vi "Drive Motors.vi"() -> ()   [LabVIEW 2018]
uses:
  <vilib>/Rock Robotics/WPI/ThirdParty/Phoenix-LabVIEW/Motor Controller/Controls/CTRE_Phoenix_MotorControl_ControlMode.ctl
  <vilib>/Rock Robotics/WPI/ThirdParty/Phoenix-LabVIEW/Motor Controller/Controls/CTRE_Phoenix_MotorControl_NeutralMode.ctl
  Framework/Robot Global Data.vi
  <vilib>/Rock Robotics/WPI/ThirdParty/Phoenix-LabVIEW/Motor Controller/Get/CTRE_Phoenix_MotorController_GetOutputCurrent_Enhanced.vi
  <vilib>/ptbypt/NI_PtbyPt.lvlib
panel:
  out "Peak Current":dbl[](array[numeric])
  in  "Target Time (s)":dbl=0.25
  in  "dropout speed":dbl=0.3
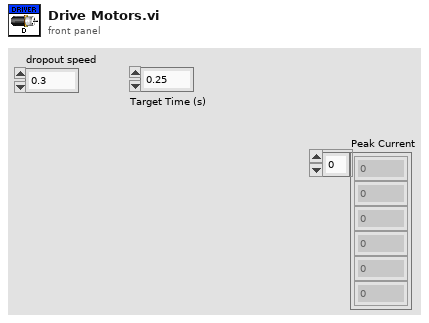
[diagram p1: front panel]
types:
  T1 = typedef "CTRE_Phoenix_MotorControl_NeutralMode.ctl" = enum8{"EEPROMSetting", "Override to Coast", "Override to Brake"}
  T2 = typedef "WPI_MotorControlDeviceRef.ctl" = cluster{"DeviceStatus":errorcluster, "Type":T3, "PWM":cluster{"PWM Channel":T4, "DeadBand":T5}, "CAN":cluster{"Device Number":u8, "SetOutput VI Ref":variant, "GetOutput VI Ref":variant, "Enable VI Ref":variant, "Disable VI Ref":variant, "Data":variant}, "Invert":bool, "DIO PWM":cluster{"PWM \"Enable\" Channel":T4, "DIOChannel":T6, "PWM Rate":dbl}}
  T3 = typedef "WPI_MotorControlType.ctl" = enum16{"PWM", "CAN", "DIO PWM"}
  T4 = typedef "FPGA_DIOPWMChannel.ctl" = enum8{"PWM 0", "PWM 1", "PWM 2", "PWM 3", "PWM 4", "PWM 5", "PWM 6", "PWM 7", "PWM 8", "PWM 9", "PWM MXP 0", "PWM MXP 1", "PWM MXP 2", "PWM MXP 3", "PWM MXP 4", "PWM MXP 5", "PWM MXP 6", "PWM MXP 7", "PWM MXP 8", "PWM MXP 9", "Invalid"}
  T5 = typedef "WPI_PWMDeadband.ctl" = cluster{"Name":string, "maxPositivePwm":i32, "minPositivePwm":i32, "centerPwm":i32, "maxNegativePwm":i32, "minNegativePwm":i32, "angularRange":u16}
  T6 = typedef "FPGA_DIOChannel.ctl" = enum8{"DIO 0", "DIO 1", "DIO 2", "DIO 3", "DIO 4", "DIO 5", "DIO 6", "DIO 7", "DIO 8", "DIO 9", "DIO MXP 0", "DIO MXP 1", "DIO MXP 2", "DIO MXP 3", "DIO MXP 4", "DIO MXP 5", "DIO MXP 6", "DIO MXP 7", "DIO MXP 8", "DIO MXP 9", "DIO MXP 10", "DIO MXP 11", "DIO MXP 12", "DIO MXP 13", "DIO MXP 14", "DIO MXP 15", "SPI Port CS1", "SPI Port CS2", "SPI Port CS3", "SPI Port MISO", "SPI Port MOSI", "Invalid"}
  T7 = typedef "CTRE_Phoenix_MotorControl_ControlMode.ctl" = u16
  T8 = typedef "WPI_DriverStationRobotMode2.ctl" = enum16{"Autonomous Disabled", "Autonomous Enabled", "Teleop Disabled", "Teleop Enabled", "Disconnected", "Finish", "Test Disabled", "Test Enabled", "Emergency Stopped"}
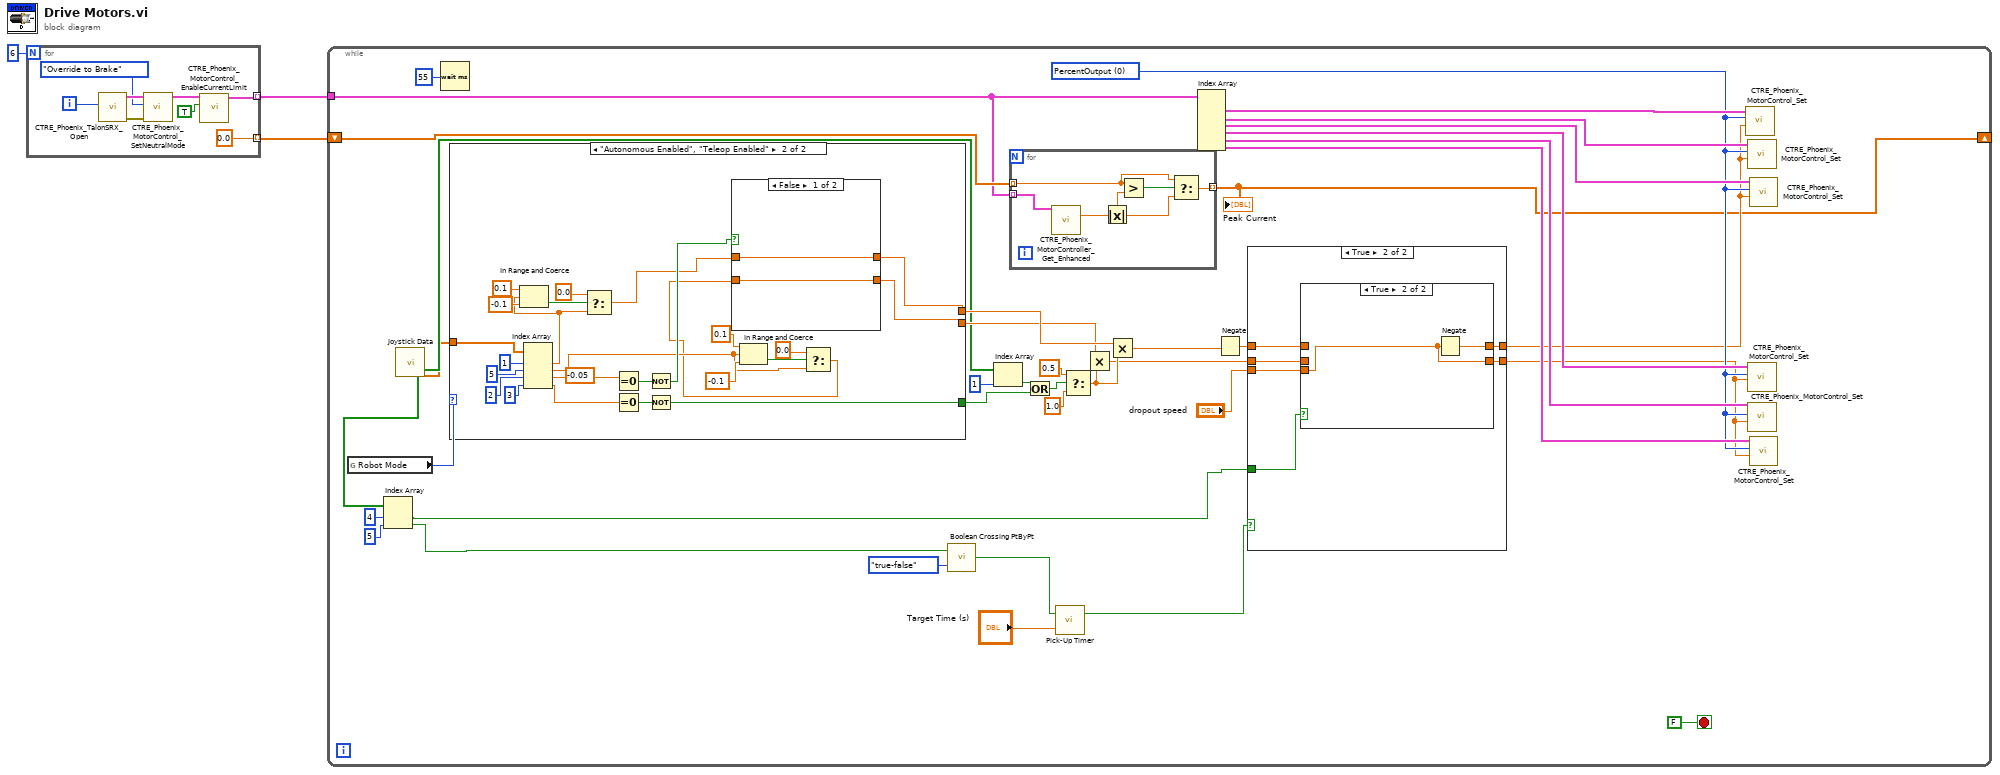
[diagram p0: block diagram]
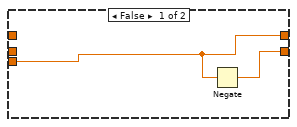
[diagram p2: hidden frame]
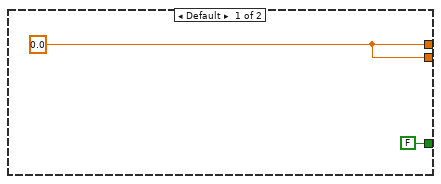
[diagram p4: hidden frame]
diagram:
  n1 = for {
    N: 6 -> [_]
    tunnel: [w6] -> w2 mode=indexing
    tunnel: [0.0] -> w1 mode=indexing
    i -> [w11]
    n2 = call <vilib>:"CTRE_Phoenix_TalonSRX_Open.vi"("Device Number"=w11) -> ("error out"=w10:errorcluster, "CAN Talon SRX Ref"=w9:T2)  [unwired: 9 in]
    n3 = call <vilib>:"CTRE_Phoenix_MotorControl_SetNeutralMode.vi"("error in (no error)"=w10, "Motor Control Neutral Mode"=CTRE_Phoenix_MotorControl_NeutralMode."Override to Brake", "PhoenixMotorControlDevRef"=w9) -> ("PhoenixMotorControlDevRef"=w7:T2)  [unwired: 7 in, 1 out]
    n4 = call <vilib>:"CTRE_Phoenix_MotorControl_EnableCurrentLimit.vi"("Enable Current Limit?"=TRUE, "PhoenixMotorControlDevRef"=w7) -> ("PhoenixMotorControlDevRef"=w6:T2)  [unwired: 8 in, 1 out]
  }
  n5 = while {
    tunnel: w2 -> [w12]
    shift-right: [w18] -> _
    shift-left: w1 -> [w19]
    stop <- FALSE stop-if-true
    w34 = T7 0 items=["PercentOutput"=0, "Position"=1, "Velocity"=2, "Current"=3, "Follower"=5, "MotionProfile"=6, "MotionMagic"=7, "MotionProfileArc"=10, "Disabled"=15] ("Control Mode")
    n6 = global read "Robot Global Data.vi" "Robot Mode"() -> (w50:T8)
    n7 = call "Joystick Data.vi"() -> ("Xbox 360 Out"=w14:bool[], "Right Buttons Out"=w26:bool[], "Xbox One Joy Out"=w25:dbl[])  [unwired: 12 in, 5 out]
    n8 = Index Array(array=w14, index #1=4 ("index"), index #2=5 ("index")) -> (element #1=w15:bool, element #2=w13:bool)
    n9 = Wait (ms)(milliseconds to wait=u32 55) -> ()  [unwired: 1 out]
    n10 = case shown="\"Autonomous Enabled\", \"Teleop Enabled\"" w50 {
      tunnel: [w70 w95] -> w42
      tunnel: [w70 w94] -> w41
      tunnel: [FALSE w85] -> w33
      tunnel: w25 -> [_ w83]
      frame Default {
        w70 = 0.0
      }
      frame "Autonomous Enabled", "Teleop Enabled" {
        (unwired) -0.05 ("lower limit")
        n11 = Index Array(array=w83, index #1=1 ("index"), index #2=5 ("index"), index #3=2 ("index"), index #4=3 ("index")) -> (element #1=w78:dbl, element #2=w72:dbl, element #3=w88:dbl, element #4=w86:dbl)
        n12 = In Range and Coerce(upper limit=0.1, x=w78, lower limit=-0.1) -> (In Range?=w80:bool)  [unwired: 1 out]
        n13 = Select(t=0.0, s=w80, f=w78) -> (s? t:f=w77:dbl)
        n14 = Equal To 0?(x=w88) -> (x = 0?=w89:bool)
        n15 = Equal To 0?(x=w86) -> (x = 0?=w87:bool)
        n16 = Not(x=w89) -> (.not. x?=w84:bool)
        n17 = Not(x=w87) -> (.not. x?=w85:bool)
        n18 = In Range and Coerce(upper limit=0.1, x=w72, lower limit=-0.1) -> (In Range?=w74:bool)  [unwired: 1 out]
        n19 = Select(t=0.0, s=w74, f=w72) -> (s? t:f=w71:dbl)
        n20 = case shown="False" w84 {
          tunnel: w71 -> [w97 w98]
          tunnel: [w96 w98] -> w95
          tunnel: [w97 w98] -> w94
          tunnel: w77 -> [w96 _]
          frame False {
          }
          frame True {
          }
        }
      }
    }
    n21 = call <vilib>:"Boolean Crossing PtByPt.vi"("direction"=enum16{"either", "false-true", "true-false"}."true-false", "input"=w13) -> ("crossing"=w22:bool)  [unwired: 1 in]
    n22 = Index Array(array=w26, index=1) -> (element=w32:bool)
    n23 = for {
      tunnel: w12 -> [w56] mode=indexing
      tunnel: w19 -> [w53] mode=indexing
      tunnel: [w51] -> w18 mode=indexing
      n24 = call-poly <vilib>:"CTRE_Phoenix_MotorController_Get_Enhanced.vi"("PhoenixMotorControlDevRef"=w56) -> ("Output Current"=w55:dbl)  [unwired: 12 in, 2 out]
      n25 = Absolute Value(x=w55) -> (abs(x)=w52:dbl)
      n26 = Greater?(x=w53, y=w52) -> (0:w54:bool)
      n27 = Select(t=w53, s=w54, f=w52) -> (s? t:f=w51:dbl)
    }
    "Peak Current" <- w18
    n28 = Or(x=w32, y=w33) -> (x .or. y?=w31:bool)
    n29 = call "Pick-Up Timer.vi"("Target Time (s)"="Target Time (s)", "Reset Timer"=w22) -> ("Time Reached?"=w21:bool)  [unwired: 1 out]
    n30 = Select(t=0.5, s=w31, f=1.0) -> (s? t:f=w40:dbl)
    n31 = Multiply(x=w41, y=w40) -> (x*y=w27:dbl)
    n32 = Multiply(x=w42, y=w40) -> (x*y=w39:dbl)
    n33 = Index Array(array=w12) -> (element #1=w49:T2, element #2=w48:T2, element #3=w35:T2, element #4=w38:T2, element #5=w37:T2, element #6=w36:T2)  [unwired: 6 in]
    n34 = Negate(x=w39) -> (-x=w29:dbl)
    n35 = case shown="True" w21 {
      tunnel: [w57 w64] -> w30
      tunnel: w29 -> [_ w63]
      tunnel: [w58 w62] -> w28
      tunnel: w27 -> [_ w61]
      tunnel: w15 -> [_ w60]
      tunnel: "dropout speed" -> [w57 w59]
      frame False {
        n36 = Negate(x=w57) -> (-x=w58:dbl)
      }
      frame True {
        n37 = case shown="True" w60 {
          tunnel: [w66 w68] -> w64
          tunnel: w63 -> [w66 _]
          tunnel: [w65 w67] -> w62
          tunnel: w61 -> [w65 _]
          tunnel: w59 -> [_ w67]
          frame False {
          }
          frame True {
            n38 = Negate(x=w67) -> (-x=w68:dbl)
          }
        }
      }
    }
    n39 = call <vilib>:"CTRE_Phoenix_MotorControl_Set.vi"("Output"=w30, "Control Mode"=w34, "PhoenixMotorControlDevRef"=w49) -> ()  [unwired: 7 in, 2 out]
    n40 = call <vilib>:"CTRE_Phoenix_MotorControl_Set.vi"("Output"=w30, "Control Mode"=w34, "PhoenixMotorControlDevRef"=w48) -> ()  [unwired: 7 in, 2 out]
    n41 = call <vilib>:"CTRE_Phoenix_MotorControl_Set.vi"("Output"=w28, "Control Mode"=w34, "PhoenixMotorControlDevRef"=w38) -> ()  [unwired: 7 in, 2 out]
    n42 = call <vilib>:"CTRE_Phoenix_MotorControl_Set.vi"("Output"=w28, "Control Mode"=w34, "PhoenixMotorControlDevRef"=w37) -> ()  [unwired: 7 in, 2 out]
    n43 = call <vilib>:"CTRE_Phoenix_MotorControl_Set.vi"("Output"=w30, "Control Mode"=w34, "PhoenixMotorControlDevRef"=w35) -> ()  [unwired: 7 in, 2 out]
    n44 = call <vilib>:"CTRE_Phoenix_MotorControl_Set.vi"("Output"=w28, "Control Mode"=w34, "PhoenixMotorControlDevRef"=w36) -> ()  [unwired: 7 in, 2 out]
  }
